vi "dfd_Maxflat Lowpass Design.vi"(6 "fs [Hz]":dbl=1.0, 7 "filter type":enum16{"IIR", "FIR", "Symmetric FIR"}(ring), 8 "error IO":errorcluster, 9 "3dB cutoff freq":dbl=0.25, 10 "denominator order":i32, 11 "numerator order":i32=10) -> (0 "error out":errorcluster, 1 "gain":dbl, 2 "poles":cdb[](array[numeric]), 3 "zeros":cdb[](array[numeric]))   [LabVIEW 2017, in "NI_DigFilter_Design.lvlib"]
uses:
  <vilib>/addons/Digital Filter Design/NI_DigFilter_Design.lvlib
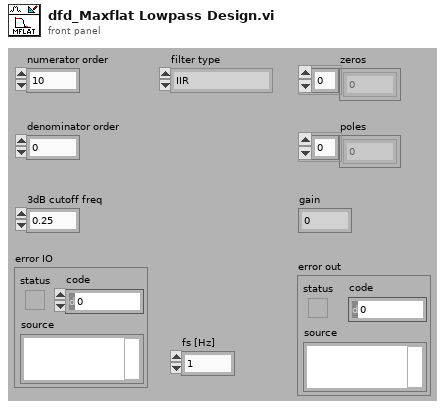
[diagram p1: front panel]
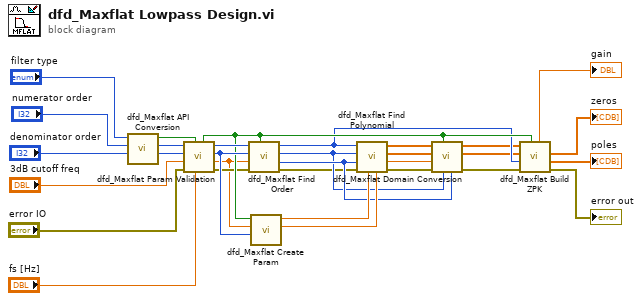
[diagram p0: block diagram]
diagram:
  n1 = call <vilib>:"dfd_Maxflat API Conversion.vi"("denominator order in"="denominator order", "numerator order in"="numerator order", "filter type"="filter type") -> ("denominator order out"=w2:i32, "numerator order out"=w4:i32, "symmetric FIR ? (T)"=w1:bool)  [unwired: 6 out]
  n2 = call <vilib>:"dfd_Maxflat Param Validation.vi"("fs"="fs [Hz]", "symmetric FIR ? (T)"=w1, "error in (no error)"="error IO", "3dB cutoff freq"="3dB cutoff freq", "denominator order"=w2, "numerator order"=w4) -> ("error out"=w15:errorcluster, "normalized fc"=w14:dbl, "dup denominator order"=w24:i32, "mod numerator order"=w25:i32, "symmetric FIR out"=w20:bool)  [unwired: 1 out]
  n3 = call <vilib>:"dfd_Maxflat Find Order.vi"("symmetric FIR ? (T)"=w20, "error in (no error)"=w15, "normalized fc"=w14, "denominator order"=w24, "numerator order"=w25) -> ("error out"=w17:errorcluster, "N"=w21:i32, "M"=w18:i32, "L"=w19:i32)  [unwired: 3 out]
  n4 = call <vilib>:"dfd_Maxflat Create Param.vi"("denominator order"=w24, "normalized fc"=w14, "symmetric FIR ? (T)"=w20) -> ("H0"=w23:dbl, "x0"=w22:dbl)  [unwired: 7 out]
  n5 = call <vilib>:"dfd_Maxflat Find Polynomial.vi"("H0"=w23, "x0"=w22, "error in (no error)"=w17, "N"=w21, "M"=w18, "L"=w19) -> ("error out"=w11:errorcluster, "c"=w13:dbl, "denominator"=w8:dbl[], "numerator"=w7:dbl[])  [unwired: 1 in, 1 out]
  n6 = call <vilib>:"dfd_Maxflat Domain Conversion.vi"("N"=w21, "M"=w18, "symmetric FIR ? (T)"=w20, "error in (no error)"=w11, "c"=w13, "denominator"=w8, "numerator"=w7) -> ("error out"=w12:errorcluster, "poles"=w10:cdb[], "zeros"=w9:cdb[])  [unwired: 2 out]
  n7 = call <vilib>:"dfd_Maxflat Build ZPK.vi"("symmetric FIR ? (T)"=w20, "error in (no error)"=w12, "L"=w19, "poles"=w10, "zeros"=w9) -> ("error out"=→"error out":errorcluster, "poles"=→"poles":cdb[], "zeros"=→"zeros":cdb[], "gain"=→"gain":dbl)  [unwired: 3 out]
